vi "GettingStarted_Acq_Tap_148X_FPGA.vi"() -> ()   [LabVIEW 2023, in "GettingStarted_Acq_Tap_148X_FPGA.lvlib"]
uses:
  GettingStarted_Acq_Tap_148X_FPGA.lvlib
  <vilib>/Platform/TimedLoop/XDataNode/XDataNode.xnode
  <vilib>/Platform/TimedLoop/XDataNode/nitl_modes.ctl
  <vilib>/Platform/TimedLoop/XDataNode/XDNodeRunTimeDep.lvlib
  <vilib>/Platform/TimedLoop/XDataNode/wakeup.ctl
  <vilib>/Platform/TimedLoop/XDataNode/timing_clust.ctl
  <instrlib>/FlexRIO/CSI-2/v2/FPGA/NI CSI-2 API FPGA v2.lvlib
  <vilib>/eio/EIONode/EIONode.xnode
  <instrlib>/FlexRIO/API/FPGA/v1/FlexRIO API FPGA v1.lvlib
  <instrlib>/_niInstr/Basic Elements/v1/FPGA/niInstr Basic Elements v1 FPGA.lvlib
  Common/GettingStarted_Common_148X_FPGA.lvlib
  <vilib>/rvi/eio/common/nirviEmuTemplateMethod_errors.vi
  <instrlib>/FlexRIO/CSI-2/v2/FPGA/Types/Channel-Based Acquistion Engine Configuration.ctl
  <instrlib>/FlexRIO/CSI-2/v2/FPGA/Types/Global Acquisition Engine Configuration.ctl
  <instrlib>/FlexRIO/CSI-2/v2/FPGA/Types/Global Acquisition Engine State.ctl
  <instrlib>/FlexRIO/CSI-2/v2/FPGA/Types/GPIO Bank.ctl
  Common/Types/SerDes Identifier.ctl
  Types/Serial Input Channel Status.ctl
  <instrlib>/FlexRIO/CSI-2/v2/FPGA/DRAM Manager/Public/Partition Range.ctl
  <instrlib>/FlexRIO/CSI-2/v2/FPGA/DRAM Manager/DRAM Manager v2.lvlib
  <instrlib>/FlexRIO/CSI-2/v2/FPGA/Types/Channel-Based Acquisition Engine State.ctl
  Common/Types/DRAM Status.ctl
  Common/Types/GPIO User Bank.ctl
  Common/Types/Display Channel Status.ctl
  <instrlib>/FlexRIO/CSI-2/v2/FPGA/Types/Display Parameters.ctl
  <instrlib>/FlexRIO/CSI-2/v2/Common/Types/LLP Data Type.ctl
  <instrlib>/FlexRIO/CSI-2/v2/Common/NI CSI-2 API Common v2.lvlib
  Types/Serial Input Channel Datapath Configuration.ctl
panel:
  in  "channel configs":T1[](array[typedef]) {"channel acq config"."first packet data type select mask" format="%.0x"; "channel acq config"."last packet data type select mask" format="%.0x"}
  in  "reset timestamp (strobe)":bool
  out "user gpio bank destination":T3
  in  "user gpio bank source":T3
  in  "gpio routes":i8[](array[numeric])=[-1, -1, -1, -1, -1, -1, -1, -1, -1, -1, -1, -1, -1, -1, -1, -1, -1, -1, -1, -1, -1, -1, -1, -1, -1, -1, -1, -1, -1, -1, -1, -1, -1, -1, -1, -1, -1, -1, -1, -1, -1, -1, -1, -1, -1, -1, -1, -1, -1, -1, -1, -1, -1, -1, -1, -1, -1, -1, -1, -1, -1, -1, -1, -1, -1, -1, -1, -1, -1, -1, -1, -1, -1, -1, -1, -1, -1, -1, -1, -1, -1, -1, -1, -1, -1, -1, -1, -1, -1, -1, -1, -1, -1, -1, -1, -1]
  out "display channel status":T4[](array[typedef])
  in  "enabled display channels":bool[](array[boolean])=[FALSE, FALSE, FALSE, FALSE, FALSE, FALSE, FALSE, FALSE]
  in  "display serial channel selectors":fxp<+,3,3>[](array[numeric])=[0.0, 0.0, 0.0, 0.0, 0.0, 0.0, 0.0, 0.0]
  in  "serial channel display parameters":T5[](array[typedef])=[{"virtual channel"=0.0, "payload data type"=enum."Frame Start", "frame skip count"=0, "line skip count"=0, "pixel skip count"=0.0}, {"virtual channel"=0.0, "payload data type"=enum."Frame Start", "frame skip count"=0, "line skip count"=0, "pixel skip count"=0.0}, {"virtual channel"=0.0, "payload data type"=enum."Frame Start", "frame skip count"=0, "line skip count"=0, "pixel skip count"=0.0}, {"virtual channel"=0.0, "payload data type"=enum."Frame Start", "frame skip count"=0, "line skip count"=0, "pixel skip count"=0.0}, {"virtual channel"=0.0, "payload data type"=enum."Frame Start", "frame skip count"=0, "line skip count"=0, "pixel skip count"=0.0}, {"virtual channel"=0.0, "payload data type"=enum."Frame Start", "frame skip count"=0, "line skip count"=0, "pixel skip count"=0.0}, {"virtual channel"=0.0, "payload data type"=enum."Frame Start", "frame skip count"=0, "line skip count"=0, "pixel skip count"=0.0}, {"virtual channel"=0.0, "payload data type"=enum."Frame Start", "frame skip count"=0, "line skip count"=0, "pixel skip count"=0.0}]
  out "serdes gpio bank input select valid":bool
  out "gpio bank input":T7
  in  "gpio bank input select":T8
  out "serdes gpio bank output select valid":bool
  in  "gpio bank\noutput enable":T7
  in  "gpio bank output select":T8
  in  "gpio bank output":T7
  out "gpio timestamp fifo overflow":bool
  out "serial input channel status":T9[](array[typedef])=[{"acq state"=enum."Idle", "stop timed out"=FALSE, "bad packet header"=FALSE, "bad packet payload"=FALSE, "bad packet size"=FALSE, "dram status"={"bytes written"=0, "bytes read"=0, "overflow"=FALSE, "partition full"=FALSE, "last byte flushed"=FALSE}}, {"acq state"=enum."Idle", "stop timed out"=FALSE, "bad packet header"=FALSE, "bad packet payload"=FALSE, "bad packet size"=FALSE, "dram status"={"bytes written"=0, "bytes read"=0, "overflow"=FALSE, "partition full"=FALSE, "last byte flushed"=FALSE}}, {"acq state"=enum."Idle", "stop timed out"=FALSE, "bad packet header"=FALSE, "bad packet payload"=FALSE, "bad packet size"=FALSE, "dram status"={"bytes written"=0, "bytes read"=0, "overflow"=FALSE, "partition full"=FALSE, "last byte flushed"=FALSE}}, {"acq state"=enum."Idle", "stop timed out"=FALSE, "bad packet header"=FALSE, "bad packet payload"=FALSE, "bad packet size"=FALSE, "dram status"={"bytes written"=0, "bytes read"=0, "overflow"=FALSE, "partition full"=FALSE, "last byte flushed"=FALSE}}, {"acq state"=enum."Idle", "stop timed out"=FALSE, "bad packet header"=FALSE, "bad packet payload"=FALSE, "bad packet size"=FALSE, "dram status"={"bytes written"=0, "bytes read"=0, "overflow"=FALSE, "partition full"=FALSE, "last byte flushed"=FALSE}}, {"acq state"=enum."Idle", "stop timed out"=FALSE, "bad packet header"=FALSE, "bad packet payload"=FALSE, "bad packet size"=FALSE, "dram status"={"bytes written"=0, "bytes read"=0, "overflow"=FALSE, "partition full"=FALSE, "last byte flushed"=FALSE}}, {"acq state"=enum."Idle", "stop timed out"=FALSE, "bad packet header"=FALSE, "bad packet payload"=FALSE, "bad packet size"=FALSE, "dram status"={"bytes written"=0, "bytes read"=0, "overflow"=FALSE, "partition full"=FALSE, "last byte flushed"=FALSE}}, {"acq state"=enum."Idle", "stop timed out"=FALSE, "bad packet header"=FALSE, "bad packet payload"=FALSE, "bad packet size"=FALSE, "dram status"={"bytes written"=0, "bytes read"=0, "overflow"=FALSE, "partition full"=FALSE, "last byte flushed"=FALSE}}]
  in  "dram partition configs":T12[](array[typedef])=[{"first address"=0, "last address"=0}, {"first address"=0, "last address"=0}, {"first address"=0, "last address"=0}, {"first address"=0, "last address"=0}, {"first address"=0, "last address"=0}, {"first address"=0, "last address"=0}, {"first address"=0, "last address"=0}, {"first address"=0, "last address"=0}]
  out "dram manager 1.num active streams":fxp<+,3,3>
  out "dram manager 0.num active streams":fxp<+,3,3>
  in  "dram arbiter config":T13={"write grant time (clocks)"=256, "read grant time (clocks)"=256}
  in  "write time slice":u16=256
  in  "request time slice":u16=256
  in  "enable sync pulse":bool
  in  "generate sync pulse (strobe)":bool
  out "global acq state":T14
  in  "global acq config":T15
  in  "sw stop trigger (strobe)":bool
  in  "sw start trigger (strobe)":bool
  in  "reset (strobe)":bool
  out "flexrio.module.dram ready 0":bool
  out "flexrio.module.io ready 0":bool
  out "flexrio.module.io error 0":i32
  out "user timestamp fifo overflow":bool
  # "Global Acquisition Configuration"
  # "Channel Configuration"
  # "GPIO Control"
  # "GPIO Routing"
  # "Display Configuration"
  # "Timestamp Synchronization"
  # "User Timestamps"
  # "DRAM Manager Configuration"
  # "Module Status"
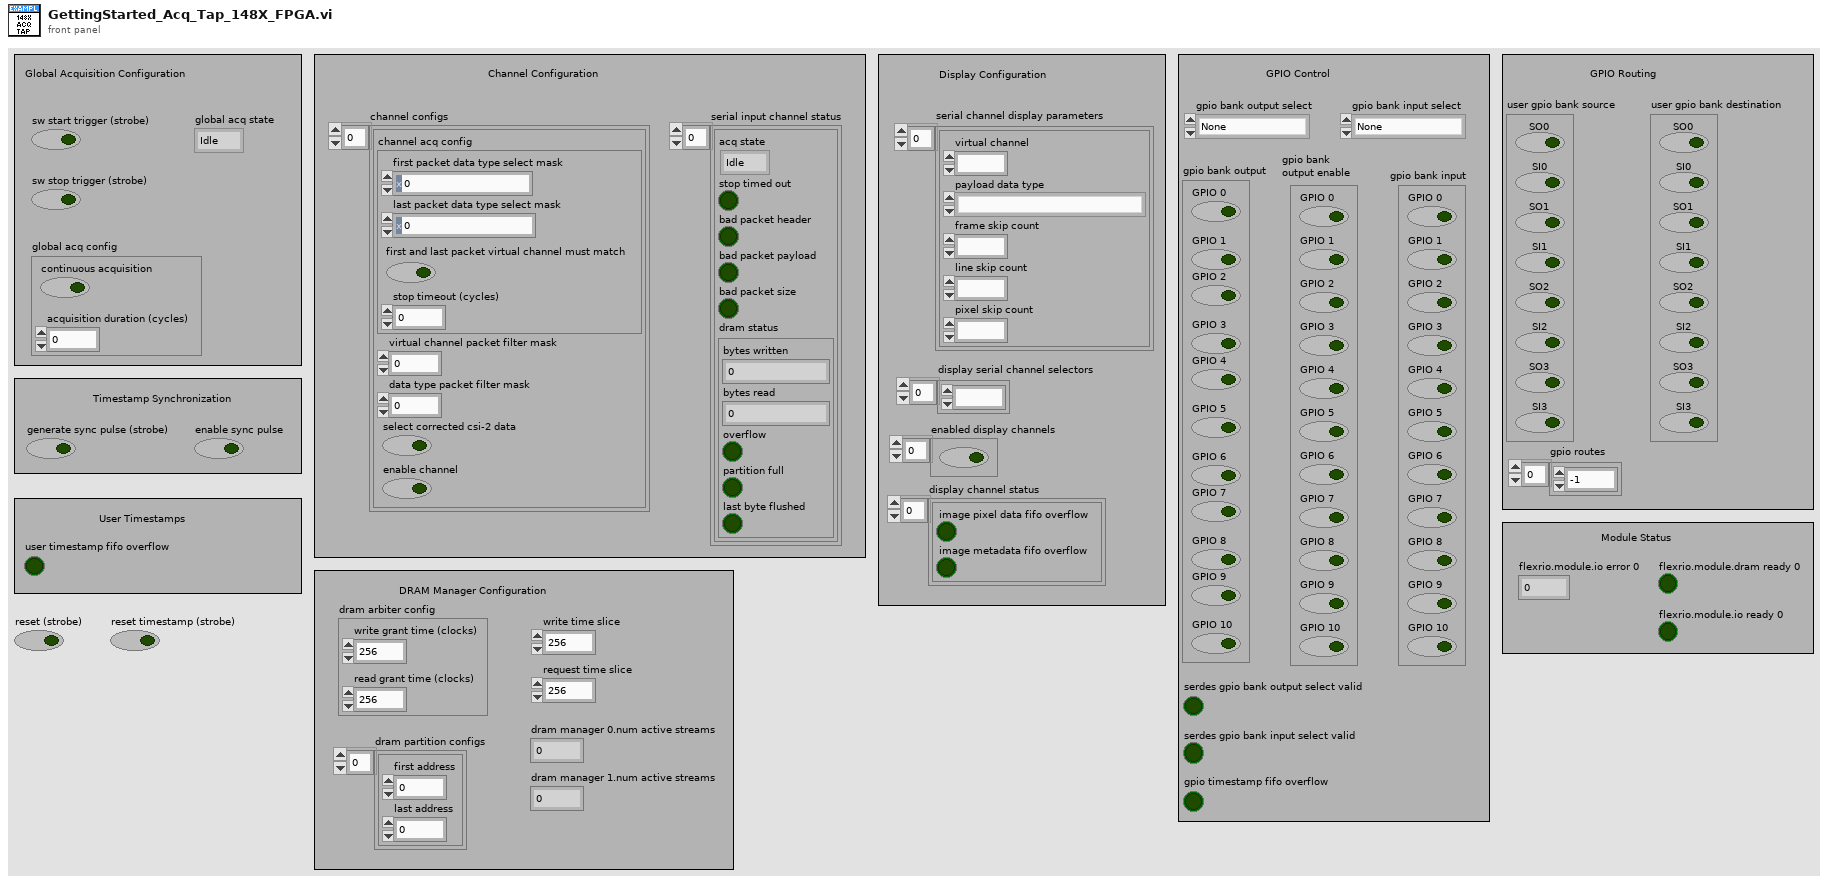
[diagram p1: front panel]
types:
  T1 = typedef "GettingStarted_Acq_Tap_148X_FPGA.lvlib/Serial Input Channel Datapath Configuration.ctl" = cluster{"channel acq config":T2, "virtual channel packet filter mask":u16, "data type packet filter mask":u64, "select corrected csi-2 data":bool, "enable channel":bool}
  T2 = typedef "NI CSI-2 API FPGA v2.lvlib/Channel-Based Acquistion Engine Configuration.ctl" = cluster{"stop timeout (cycles)":u32, "first packet data type select mask":u64, "last packet data type select mask":u64, "first and last packet virtual channel must match":bool}
  T3 = typedef "GettingStarted_Common_148X_FPGA.lvlib/GPIO User Bank.ctl" = cluster{"SO0":bool, "SI0":bool, "SO1":bool, "SI1":bool, "SO2":bool, "SI2":bool, "SO3":bool, "SI3":bool}
  T4 = typedef "GettingStarted_Common_148X_FPGA.lvlib/Display Channel Status.ctl" = cluster{"image pixel data fifo overflow":bool, "image metadata fifo overflow":bool}
  T5 = typedef "NI CSI-2 API FPGA v2.lvlib/Display Parameters.ctl" = cluster{"virtual channel":fxp<+,4,4>, "payload data type":T6, "frame skip count":u16, "line skip count":u8, "pixel skip count":fxp<+,5,5>}
  T6 = typedef "NI CSI-2 API Common v2.lvlib/LLP Data Type.ctl" = enum8{"Frame Start", "Frame End", "Line Start", "Line End", "End of Transmission", "Reserved 0", "Reserved 1", "Reserved 2", "Generic Short Packet 1", "Generic Short Packet 2", "Generic Short Packet 3", "Generic Short Packet 4", "Generic Short Packet 5", "Generic Short Packet 6", "Generic Short Packet 7", "Generic Short Packet 8", "Null", "Blanking Data", "Embedded 8-bit non Image Data", "Generic Long Packet 1", "Generic Long Packet 2", "Generic Long Packet 3", "Generic Long Packet 4", "Reserved 3", "YUV420 8-bit", "YUV420 10-bit", "Legacy YUV420 8-bit", "Reserved 4", "YUV420 8-bit Chroma Shifted", "YUV420 10-bit Chroma Shifted", "YUV422 8-bit", "YUV422 10-bit", "RGB444", "RGB555", "RGB565", "RGB666", "RGB888", "Reserved 5", "Reserved 6", "RAW 24", "RAW 6", "RAW 7", "RAW 8", "RAW 10", "RAW 12", "RAW 14", "RAW 16", "RAW 20", "User Defined 8-bit Data 1", "User Defined 8-bit Data 2", "User Defined 8-bit Data 3", "User Defined 8-bit Data 4", "User Defined 8-bit Data 5", "User Defined 8-bit Data 6", "User Defined 8-bit Data 7", "User Defined 8-bit Data 8", "USL Command", "Reserved 7", "Reserved 8", "Reserved 9", "Reserved 10", "Reserved 11", "Reserved 12", "LRTE EPD Spacer"}
  T7 = typedef "NI CSI-2 API FPGA v2.lvlib/GPIO Bank.ctl" = cluster{"GPIO 0":bool, "GPIO 1":bool, "GPIO 2":bool, "GPIO 3":bool, "GPIO 4":bool, "GPIO 5":bool, "GPIO 6":bool, "GPIO 7":bool, "GPIO 8":bool, "GPIO 9":bool, "GPIO 10":bool}
  T8 = typedef "GettingStarted_Common_148X_FPGA.lvlib/SerDes Identifier.ctl" = enum8{"None", "SI 0 Deserializer", "SI 1 Deserializer", "SI 2 Deserializer", "SI 3 Deserializer", "SI 4 Deserializer", "SI 5 Deserializer", "SI 6 Deserializer", "SI 7 Deserializer", "SO 0 Serializer", "SO 1 Serializer", "SO 2 Serializer", "SO 3 Serializer", "SO 4 Serializer", "SO 5 Serializer", "SO 6 Serializer", "SO 7 Serializer", "SI 0 SI 1 Deserializer", "SI 2 SI 3 Deserializer", "SI 4 SI 5 Deserializer", "SI 6 SI 7 Deserializer"}
  T9 = typedef "GettingStarted_Acq_Tap_148X_FPGA.lvlib/Serial Input Channel Status.ctl" = cluster{"acq state":T10, "stop timed out":bool, "bad packet header":bool, "bad packet payload":bool, "bad packet size":bool, "dram status":T11}
  T10 = typedef "NI CSI-2 API FPGA v2.lvlib/Channel-Based Acquisition Engine State.ctl" = enum8{"Idle", "Wait for First Packet Header", "Acquire", "Wait for Last Packet Header", "Wait for End of Last Packet"}
  T11 = typedef "GettingStarted_Common_148X_FPGA.lvlib/DRAM Status.ctl" = cluster{"bytes written":u64, "bytes read":u64, "overflow":bool, "partition full":bool, "last byte flushed":bool}
  T12 = typedef "DRAM Manager v2.lvlib/Partition Range.ctl" = cluster{"first address":u32, "last address":u32}
  T13 = cluster{"write grant time (clocks)":u16, "read grant time (clocks)":u16}
  T14 = typedef "NI CSI-2 API FPGA v2.lvlib/Global Acquisition Engine State.ctl" = enum8{"Idle", "Ready For Start Trigger", "Acquire", "Error"}
  T15 = typedef "NI CSI-2 API FPGA v2.lvlib/Global Acquisition Engine Configuration.ctl" = cluster{"continuous acquisition":bool, "acquisition duration (cycles)":u64}
  T16 = typedef "GettingStarted_Common_148X_FPGA.lvlib/Common Resources.ctl" = cluster{"sync pulse resources":T17, "serial channel resources":T18, "dram manager 0":T20, "dram manager 1":T20}
  T17 = typedef "NI CSI-2 API FPGA v2.lvlib/Sync Pulse Resources.ctl" = cluster{"sync pulse destination terminal":refnum<k21>, "sync100":refnum<k21>, "sync pulse source terminal":refnum<k21>, "imported sync pulse register":refnum<k21>, "generate sync pulse handshake":refnum<k21>, "enable sync pulse register":refnum<k21>, "sync pulse clock":refnum<k21>}
  T18 = typedef "GettingStarted_Common_148X_FPGA.lvlib/Serial Channel Resources.ctl" = cluster{"sc 0":T19, "sc 1":T19, "sc 2":T19, "sc 3":T19, "sc 4":T19, "sc 5":T19, "sc 6":T19, "sc 7":T19}
  T19 = typedef "GettingStarted_Common_148X_FPGA.lvlib/Single Serial Channel Resources.ctl" = cluster{"completed frames register":refnum<k21>}
  T20 = typedef "DRAM Manager v2.lvlib/DRAM Manager.ctl" = cluster{"DRAM class":refnum<class "niInstr Memory DRAM v1 FPGA.lvclass">, "process clock":refnum<k21>, "registers":T21, "FIFOs":T23, "num active streams":fxp<+,3,3>, "max open read requests":u16}
  T21 = typedef "DRAM Manager v2.lvlib/DRAM Manager Registers.ctl" = cluster{"configuration":cluster{"write time slice":refnum<k21>, "request time slice":refnum<k21>, "DRAM arbiter config":refnum<k21>, "partition config":refnum<k21>}, "reset":cluster{"handshake":T22, "process":cluster{"in":refnum<k21>, "out":refnum<k21>}, "write":cluster{"in":refnum<k21>, "out 0":refnum<k21>, "out 1":refnum<k21>, "out 2":refnum<k21>, "out 3":refnum<k21>}, "read":cluster{"in":refnum<k21>, "out 0":refnum<k21>, "out 1":refnum<k21>, "out 2":refnum<k21>, "out 3":refnum<k21>}}, "status":cluster{"partition full":refnum<k21>}}
  T22 = typedef "DRAM Manager v2.lvlib/Handshake Registers.ctl" = cluster{"start.go":refnum<k21>, "start.go rcvd":refnum<k21>, "done.go":refnum<k21>, "done.go rcvd":refnum<k21>}
  T23 = typedef "DRAM Manager v2.lvlib/DRAM Manager FIFOs.ctl" = cluster{"write data":cluster{"FIFO 0":T24, "FIFO 1":T24, "FIFO 2":T24, "FIFO 3":T24}, "request metadata":cluster{"FIFO":T25}, "read data VOQ":cluster{"FIFO 0":T26, "FIFO 1":T26, "FIFO 2":T26, "FIFO 3":T26}, "read data":cluster{"FIFO 0":T26, "FIFO 1":T26, "FIFO 2":T26, "FIFO 3":T26}}
  T24 = typedef "DRAM Manager v2.lvlib/Write Data FIFO Ref.ctl" = refnum<k21>
  T25 = typedef "DRAM Manager v2.lvlib/Read Request Metadata FIFO Ref.ctl" = refnum<k21>
  T26 = typedef "DRAM Manager v2.lvlib/Read Data FIFO Ref.ctl" = refnum<k21>
  T27 = typedef "XDNodeRunTimeDep.lvlib/timing_clust.ctl" = cluster{"Expected End [f-1]":u64, "Actual End [f-1]":u64, "Finished Late? [f-1]":bool, "Expected End [i-1]":u64, "Actual End [i-1]":u64, "Finished Late? [i-1]":bool, "Expected Start [i]":u64, "Actual Start [i]":u64, "Expected Start [f]":u64, "Actual Start [f]":u64, "Source Name":string, "Structure Name":string, "Period":i64, "Deadline":i64, "Offset":i64, "Start":i64, "Priority":i32, "Timeout":i32, "Mode":T28, "Wakeup Reason":T29, "Error":errorcluster, "Source Type":string, "Secondary Source Type":string, "Global End Time":u64, "Global Start Time":u64, "Frame Duration":u64, "Iteration Duration":u64, "Assigned CPU":i32, "I/O Scan Engine Mode":u32}
  T28 = typedef "XDNodeRunTimeDep.lvlib/nitl_modes.ctl" = enum32{"No Change", "Process missed periods, maintain original phase", "Discard missed periods, maintain original phase", "Process missed periods, ignore original phase", "Discard missed periods, ignore original phase"}
  T29 = typedef "XDNodeRunTimeDep.lvlib/wakeup.ctl" = enum32{"Normal", "Aborted", "Asynchronous wakeup", "Timing source error", "Timed loop error", "Timeout"}
  T30 = typedef "GettingStarted_Common_148X_FPGA.lvlib/GPIO Bank Output Configuration.ctl" = cluster{"gpio bank":T7, "gpio bank output enable":T7}
  T31 = typedef "NI CSI-2 API FPGA v2.lvlib/Timestamp Counter Value.ctl" = cluster{"counter value":u64, "valid":bool}
  T32 = typedef "GettingStarted_Common_148X_FPGA.lvlib/Tagged LLP Packets Cluster.ctl" = cluster{"tagged llp packet 0":T33, "tagged llp packet 1":T33, "tagged llp packet 2":T33, "tagged llp packet 3":T33, "tagged llp packet 4":T33, "tagged llp packet 5":T33, "tagged llp packet 6":T33, "tagged llp packet 7":T33}
  T33 = typedef "NI CSI-2 API FPGA v2.lvlib/Tagged LLP Packet.ctl" = cluster{"tag":T34, "llp packet":T38}
  T34 = typedef "NI CSI-2 API FPGA v2.lvlib/FPGA LLP Packet Tag.ctl" = cluster{"timestamp":T35, "size":T37}
  T35 = typedef "NI CSI-2 API FPGA v2.lvlib/FPGA LLP Packet Timestamp.ctl" = cluster{"valid":bool, "count":fxp<+,50,50>, "id":T36, "metadata":u8}
  T36 = typedef "NI CSI-2 API FPGA v2.lvlib/Timestamp ID.ctl" = enum8{"SI0 LLP", "SI1 LLP", "SI2 LLP", "SI3 LLP", "SI4 LLP", "SI5 LLP", "SI6 LLP", "SI7 LLP", "SO0 LLP", "SO1 LLP", "SO2 LLP", "SO3 LLP", "SO4 LLP", "SO5 LLP", "SO6 LLP", "SO7 LLP", "Ser0 GPIO Bank", "Ser1 GPIO Bank", "Ser2 GPIO Bank", "Ser3 GPIO Bank", "Ser4 GPIO Bank", "Ser5 GPIO Bank", "Ser6 GPIO Bank", "Ser7 GPIO Bank", "Des0 GPIO Bank", "Des1 GPIO Bank", "Des2 GPIO Bank", "Des3 GPIO Bank", "Des4 GPIO Bank", "Des5 GPIO Bank", "Des6 GPIO Bank", "Des7 GPIO Bank", "User0", "User1", "User2", "User3", "User4", "User5", "User6", "User7", "User8", "User9", "User10", "User11", "User12", "User13", "User14", "User15", "User16", "User17", "User18", "User19", "User20", "User21", "User22", "User23", "User24", "User25", "User26", "User27", "User28", "User29", "User30", "User31"}
  T37 = typedef "NI CSI-2 API FPGA v2.lvlib/FPGA LLP Packet Size.ctl" = cluster{"bytes":fxp<+,17,17>, "valid":bool}
  T38 = typedef "NI CSI-2 API FPGA v2.lvlib/LLP Packet.ctl" = cluster{"header":T39, "header valid":bool, "payload":T40, "payload valid":bool, "footer":T41, "footer valid":bool, "end of packet":bool}
  T39 = typedef "NI CSI-2 API FPGA v2.lvlib/LLP Packet Header.ctl" = cluster{"word count":u16, "ecc":fxp<+,6,6>, "vcx":fxp<+,2,2>, "data type":fxp<+,6,6>, "vc":fxp<+,2,2>}
  T40 = typedef "NI CSI-2 API FPGA v2.lvlib/LLP Packet Payload.ctl" = cluster{"end of payload":bool, "end of payload index":fxp<+,3,3>, "payload data":u8[]}
  T41 = typedef "NI CSI-2 API FPGA v2.lvlib/LLP Packet Footer.ctl" = cluster{"crc":u16}
  T42 = typedef "FlexRIO 148x FPGA v1.lvlib/i2c monitor.ctl" = cluster{"monitor word":u8, "is header?":bool, "read/write_n":bool, "ack":bool, "start":bool, "stop":bool, "valid":bool}
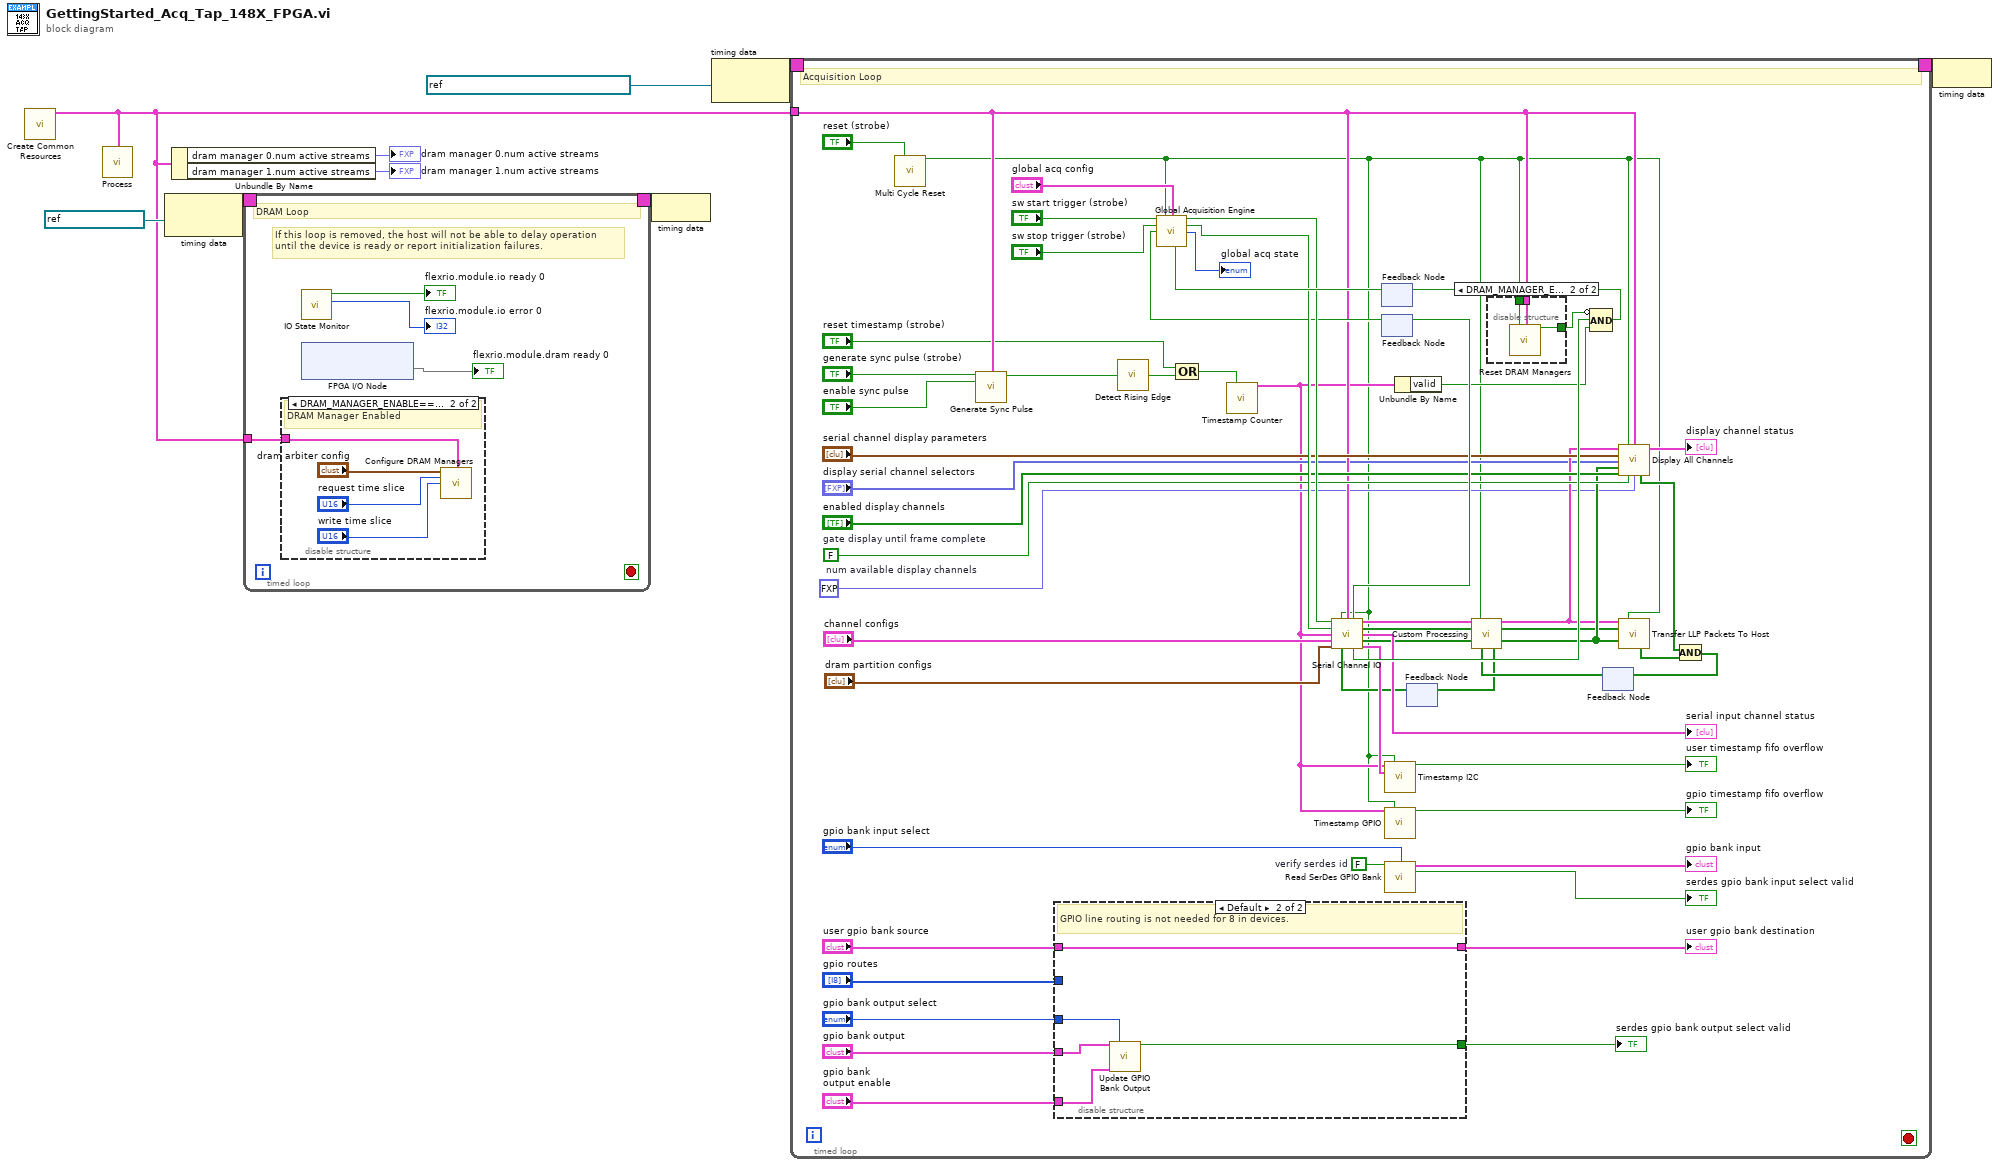
[diagram p0: block diagram]
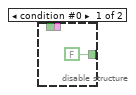
[diagram p2: hidden frame]
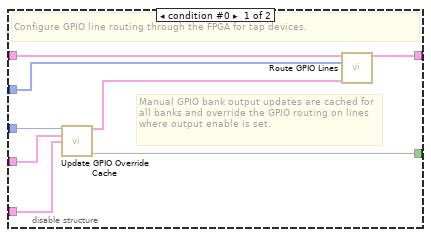
[diagram p3: hidden frame]
diagram:
  n1 = call "Create Common Resources.vi"() -> ("common resources"=w1:T16)  [unwired: 15 in]
  n2 = call "Process.vi"("resources"=w1) -> ()  [unwired: 15 in]
  n3 = node-c288(refnum<k21> "80 MHz Clock" ("Source Name")) -> (w6:T27)
  n4 = Unbundle By Name(w1) -> ("dram manager 0.num active streams"=→"dram manager 0.num active streams":fxp<+,3,3>, "dram manager 1.num active streams"=→"dram manager 1.num active streams":fxp<+,3,3>)
  n5 = timed-loop {
    timing: w6 -> [_]
    timing-out: [_] -> w5
    tunnel: w1 -> [w11]
    stop <- _ stop-if-true
    # "If this loop is removed, the host will not be able to delay operation \nuntil the device is ready or report initialization failures."
    # "DRAM Loop"
    n6 = disable-structure shown="DRAM_MANAGER_ENABLE==1, Default" {
      disable-tunnel: w11 -> [_ w17]
      frame condition #0 {
        # "DRAM Manger Disabled"
      }
      frame condition #1 (active) {
        # "DRAM Manager Enabled"
        n7 = call "Configure DRAM Managers.vi"("dram arbiter config"="dram arbiter config", "resources"=w17, "request time slice"="request time slice", "write time slice"="write time slice") -> ()  [unwired: 12 in]
      }
    }
    n8 = call <instrlib>:"IO State Monitor.vi"() -> ("flexrio.module.io error 0"=→"flexrio.module.io error 0":i32, "flexrio.module.io ready 0"=→"flexrio.module.io ready 0":bool)  [unwired: 10 in]
    n9 = xnode "FPGA I/O Node"() -> ("DRAM Ready"=→"flexrio.module.dram ready 0")  [unwired: 1 in, 1 out]
  }
  n10 = node-c288(w5) -> ()
  n11 = node-c288(refnum<k21> "IO Socket\\CSI-2 AXI Stream Clock" ("Source Name")) -> (w9:T27)
  n12 = timed-loop {
    timing: w9 -> [_]
    timing-out: [_] -> w8
    tunnel: w1 -> [w37]
    stop <- _ stop-if-true
    w25 = fxp<+,4,4> 2.0  # num available display channels
    w42 = FALSE  # gate display until frame complete
    w58 = FALSE  # verify serdes id
    # "Acquisition Loop"
    n13 = call "Multi Cycle Reset.vi"("reset (strobe)"="reset (strobe)") -> ("reset (fanout)"=w20:bool)  [unwired: 14 in]
    n14 = call "Generate Sync Pulse.vi"("generate sync pulse (strobe)"="generate sync pulse (strobe)", "resources"=w37, "enable sync pulse"="enable sync pulse") -> ("sync pulse out"=w69:bool)  [unwired: 12 in]
    n15 = disable-structure shown="Default" {
      disable-tunnel: [w89 w94] -> w54
      disable-tunnel: "user gpio bank source" -> [w88 w94]
      disable-tunnel: "gpio bank\noutput enable" -> [w82 w92]
      disable-tunnel: "gpio bank output" -> [w83 w93]
      disable-tunnel: [w86 w90] -> w50
      disable-tunnel: "gpio bank output select" -> [w84 w91]
      disable-tunnel: "gpio routes" -> [w87 _]
      frame condition #0 {
        # "Manual GPIO bank output updates are cached for all banks and override the GPIO routing on lines where output enable is set."
        # "Configure GPIO line routing through the FPGA for tap devices."
        n16 = call "Update GPIO Override Cache.vi"("override gpio bank serdes id"=w84, "override gpio bank"=w83, "override gpio bank output enable"=w82) -> ("gpio override cache"=w85:T30[], "valid override serdes id"=w86:bool)  [unwired: 11 in]
        n17 = call "Route GPIO Lines.vi"("user gpio bank in"=w88, "gpio routes"=w87, "override gpio bank ouptut configs"=w85) -> ("user gpio bank out"=w89:T3)  [unwired: 12 in]
      }
      frame condition #1 (active) {
        # "GPIO line routing is not needed for 8 in devices."
        n18 = call "Update GPIO Bank Output.vi"("gpio bank"=w93, "gpio bank serdes id"=w91, "gpio bank output enable"=w92) -> ("serdes id valid"=w90:bool)  [unwired: 12 in]
      }
    }
    "user gpio bank destination" <- w54
    "serdes gpio bank output select valid" <- w50
    n19 = call <instrlib>:"Detect Rising Edge.vi"("signal"=w69) -> ("edge detected"=w66:bool)  [unwired: 14 in]
    n20 = Compound Arithmetic op=OR("reset timestamp (strobe)", w66) -> (w72:bool)
    n21 = call <instrlib>:"Timestamp Counter.vi"("reset and start"=w72) -> ("timestamp counter value"=w23:T31)  [unwired: 14 in]
    n22 = feedback #1() -> (w75:bool)  [unwired: 1 in]
    n23 = feedback #2() -> (w61:bool)  [unwired: 1 in]
    n24 = call <instrlib>:"Global Acquisition Engine.vi"("start trigger"="sw start trigger (strobe)", "reset"=w20, "configuration"="global acq config", "stop trigger"="sw stop trigger (strobe)", "error detected"=w61, "ready for arm"=w75) -> ("arm"=w65:bool, "stop"=w64:bool, "state"=→"global acq state":T14)  [unwired: 7 in]
    n25 = call "Timestamp GPIO.vi"("timestamp counter value"=w23, "reset"=w20) -> ("gpio timestamp fifo overflow"=→"gpio timestamp fifo overflow":bool)  [unwired: 13 in]
    n26 = call "Read SerDes GPIO Bank.vi"("verify serdes id"=w58, "serdes id"="gpio bank input select") -> ("gpio bank input"=→"gpio bank input":T7, "serdes id valid"=→"serdes gpio bank input select valid":bool)  [unwired: 12 in]
    n27 = Unbundle By Name(w23) -> ("valid"=w22:bool)
    n28 = feedback #3() -> (w28:bool[])  [unwired: 1 in]
    n29 = call "Serial Channel IO.vi"("arm"=w65, "reset"=w20, "common resources"=w37, "stop"=w64, "timestamp counter value"=w23, "channel configs"="channel configs", "dram partition configs"="dram partition configs", "ready for output"=w28) -> ("acquisition error"=w47:bool, "tagged llp packets cluster"=w36:T32, "end of data"=w32:bool[], "serial input channel status"=→"serial input channel status":T9[], "tagged llp packet valid"=w35:bool[], "ready for arm"=w56:bool, "i2c monitor array"=w46:T42[])  [unwired: 1 in]
    n30 = feedback-in #2(w47) -> ()
    n31 = call "Timestamp I2C.vi"("timestamp counter value"=w23, "reset"=w20, "i2c monitor array"=w46) -> ("user timestamp fifo overflow"=→"user timestamp fifo overflow":bool)  [unwired: 12 in]
    n32 = disable-structure shown="DRAM_MANAGER_ENABLE==1, Default" {
      disable-tunnel: [FALSE ("in reset") w81] -> w68
      disable-tunnel: w37 -> [_ w80]
      disable-tunnel: w20 -> [_ w79]
      frame condition #0 {
      }
      frame condition #1 (active) {
        n33 = call "Reset DRAM Managers.vi"("reset"=w79, "resources"=w80) -> ("in reset"=w81:bool)  [unwired: 13 in]
      }
    }
    n34 = Compound Arithmetic op=AND(invert w68, w56, w22) -> (w67:bool)
    n35 = feedback-in #1(w67) -> ()
    n36 = feedback #4() -> (w30:bool[])  [unwired: 1 in]
    n37 = call "Custom Processing.vi"("tagged llp packets cluster in"=w36, "reset"=w20, "end of data in"=w32, "input valid"=w35, "ready for output"=w30) -> ("tagged llp packets cluster out"=w33:T32, "end of data out"=w31:bool[], "output valid"=w34:bool[], "ready for input"=w29:bool[])  [unwired: 7 in]
    n38 = feedback-in #3(w29) -> ()
    n39 = call "Display All Channels.vi"("tagged llp packets cluster"=w33, "reset"=w20, "common resources"=w37, "serial channel display parameters"="serial channel display parameters", "display serial channel selectors"="display serial channel selectors", "input valid"=w34, "enabled display channels"="enabled display channels", "gate display until frame complete"=w42, "num available display channels"=w25) -> ("display channel status"=→"display channel status":T4[], "ready for input"=w39:bool[])  [unwired: 5 in]
    n40 = call "Transfer LLP Packets To Host.vi"("tagged llp packets cluster"=w33, "reset"=w20, "end of data"=w31, "tagged llp packet valid"=w34) -> ("ready for input"=w40:bool[])  [unwired: 11 in]
    n41 = Compound Arithmetic op=AND(w39, w40) -> (w38:bool[])
    n42 = feedback-in #4(w38) -> ()
  }
  n43 = node-c288(w8) -> ()
